vi "add channel to configuration.vi"(8 "error in":errorcluster, 10 "channel":refnum<class "TBM channel.lvclass">, 11 "tag select module configuration in":refnum<class "tag select module configuration.lvclass">) -> (0 "error out":errorcluster, 3 "tag select module configuration out":refnum<class "tag select module configuration.lvclass">)   [LabVIEW 2013]
uses:
  tag select module configuration.lvclass
  <vilib>/NI/Tag Bus/tag/tag descriptor.lvclass
  <vilib>/NI/Tag Bus Module Framework/channel/TBM channel.lvclass
  tag select configuration.ctl
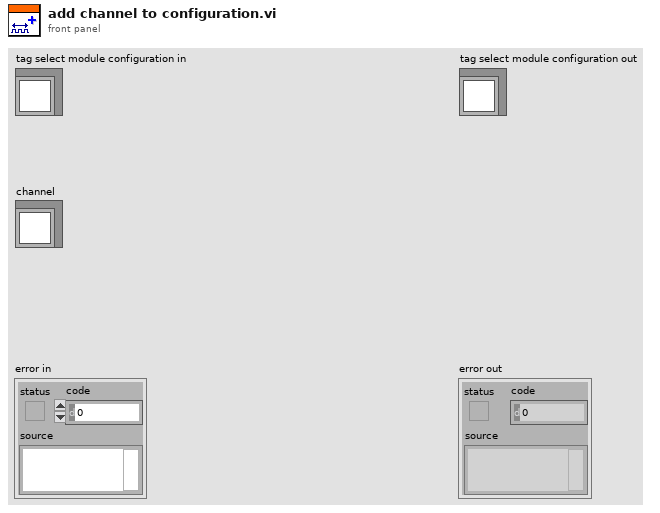
[diagram p1: front panel]
types:
  T1 = typedef "tag select module configuration.lvclass/tag select configuration.ctl" = cluster{"tag select name":string, "output":refnum<class "TBM channel.lvclass">, "select":refnum<class "TBM channel.lvclass">, "input channels":refnum<class "TBM channel.lvclass">[]}
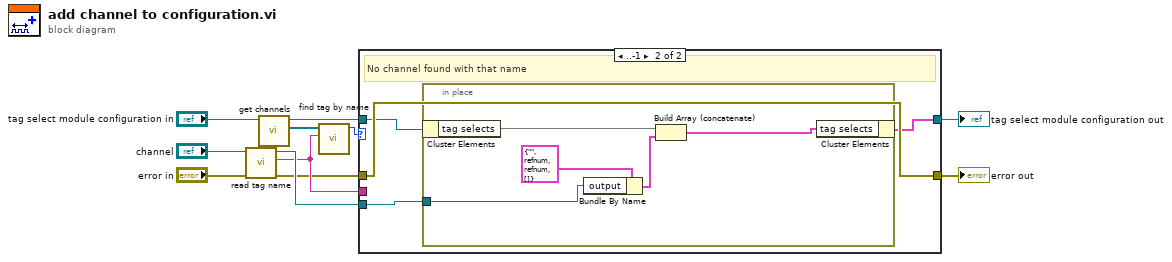
[diagram p0: block diagram]
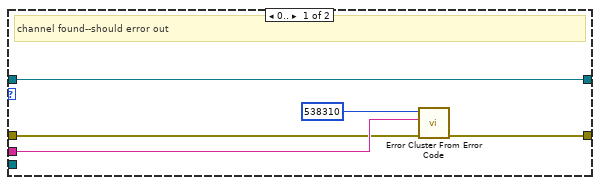
[diagram p2: hidden frame]
diagram:
  n1 = call <vilib>:"read tag name.vi"("error in"="error in", "system tag in"="channel") -> ("error out"=w2:errorcluster, "name"=w3:string, "system tag out"=w10:refnum<class "TBM channel.lvclass">)  [unwired: 7 in]
  n2 = call-dynamic "get channels.vi"("alarms module configuration in"="tag select module configuration in") -> ("channels"=w5:refnum<class "TBM channel.lvclass">[], "alarms module configuration out"=w11:refnum<class "tag select module configuration.lvclass">)  [unwired: 9 in]
  n3 = call <vilib>:"find tag by name.vi"("name"=w3, "tags in"=w5) -> ("index"=w4:i32)  [unwired: 9 in]
  n4 = case shown="..-1" w4 {
    tunnel: [w16 w19] -> w8
    tunnel: w3 -> [w14 _]
    tunnel: w2 -> [w13 w19]
    tunnel: w11 -> [w12 w17]
    tunnel: w10 -> [_ w20]
    tunnel: [w12 w18] -> w7
    frame 0.. {
      # "channel found--should error out"
      n5 = call <vilib>:"Error Cluster From Error Code.vi"("error in (no error)"=w13, "error message (\"\")"=w14, "error code (0)"=538310) -> ("error out"=w16:errorcluster)  [unwired: 6 in]
    }
    frame ..-1 {
      # "No channel found with that name"
      n6 = in-place {
        in-place-border: w20 -> [w22]
        n7 = in-place-cluster #1(w17) -> ("tag selects"=w25)
        n8 = Bundle By Name(cluster=T1 {"tag select name"="", "output"=refnum, "select"=refnum, "input channels"=[]} ("tag select config"), "output"=w22) -> (w21:T1)
        n9 = Build Array (concatenate)(w25, w21) -> (w24:T1[])
        n10 = in-place-cluster #1("tag selects"=w24) -> (w18:cluster{})
      }
    }
  }
  "error out" <- w8
  "tag select module configuration out" <- w7
